vi "Install Dependencies.vi"(7 "Stored Install Data":path, 10 "Variant":variant) -> (0 "Error Out":errorcluster)   [LabVIEW 2020, in "LMH-Toolbox.lvlib" / "LMH-Installer Tools.lvlib"]
uses:
  LMH-Installer Tools.lvlib
  Private/Type Defs/Deps State.ctl
  <vilib>/Utility/file.llb/Read From Spreadsheet File (string).vi
  LMH-Toolbox.lvlib
panel:
  out "Tab Control":T1(tab)
  out "Package Name":string
  in  "Listbox":i32(listbox)
  in  "Info Cancel Button":bool
  in  "Info Next Button":bool
  out "Status":string
  out "Download Progress":u8(slide) scale=0.0..100.0
  in  "Multicolumn Listbox":i32(listbox)
  in  "Install Next":bool
  in  "Install Cancel":bool
  in  "Summary Finish":bool
  # "Testing Dependencies . . ."
  # "Select dependencies you want to install."
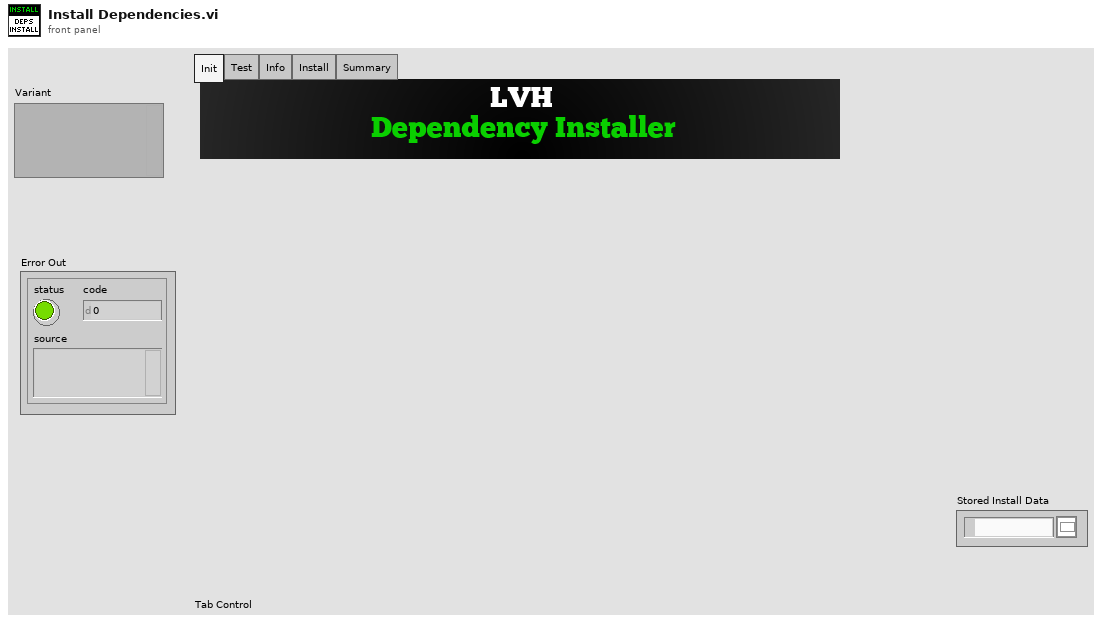
[diagram p1: front panel]
types:
  T1 = enum32{"Init", "Test", "Info", "Install", "Summary"}
  T2 = typedef "LMH-Toolbox.lvlib/LMH-Installer Tools.lvlib/Deps State.ctl" = enum16{"Init", "Test", "Info", "Install", "Summary"}
  T3 = typedef "LMH-Toolbox.lvlib/LMH-Installer Tools.lvlib/Dependency Config.ctl" = cluster{"Dependencies":T4[], "Files Installed":path[], "Dependency Config":path, "Installer Helper":path, "Dep Index":i32, "Download":T5}
  T4 = typedef "LMH-Toolbox.lvlib/LMH-Installer Tools.lvlib/Dependecy.ctl" = cluster{"Name":string, "Version":string, "Test VI Path":path, "Source URL":string, "Dep Met?":bool, "Install?":bool, "Installer Args":string}
  T5 = typedef "LMH-Toolbox.lvlib/LMH-Web.lvlib/Download Task.ctl" = cluster{"URL":string, "Local Path":path, "Download Worker":refnum<vi>, "Total Size (Bytes)":u64, "Prev Downloaded Size":u64, "Prev Download Time Stamp":timestamp}
  T6 = enum16{"Init", "Start DL", "Downloading", "DL Complete", "Done"}
  T7 = typedef "LVPoint32TypeDef.ctl" = cluster{"Horizontal":i32, "Vertical":i32}
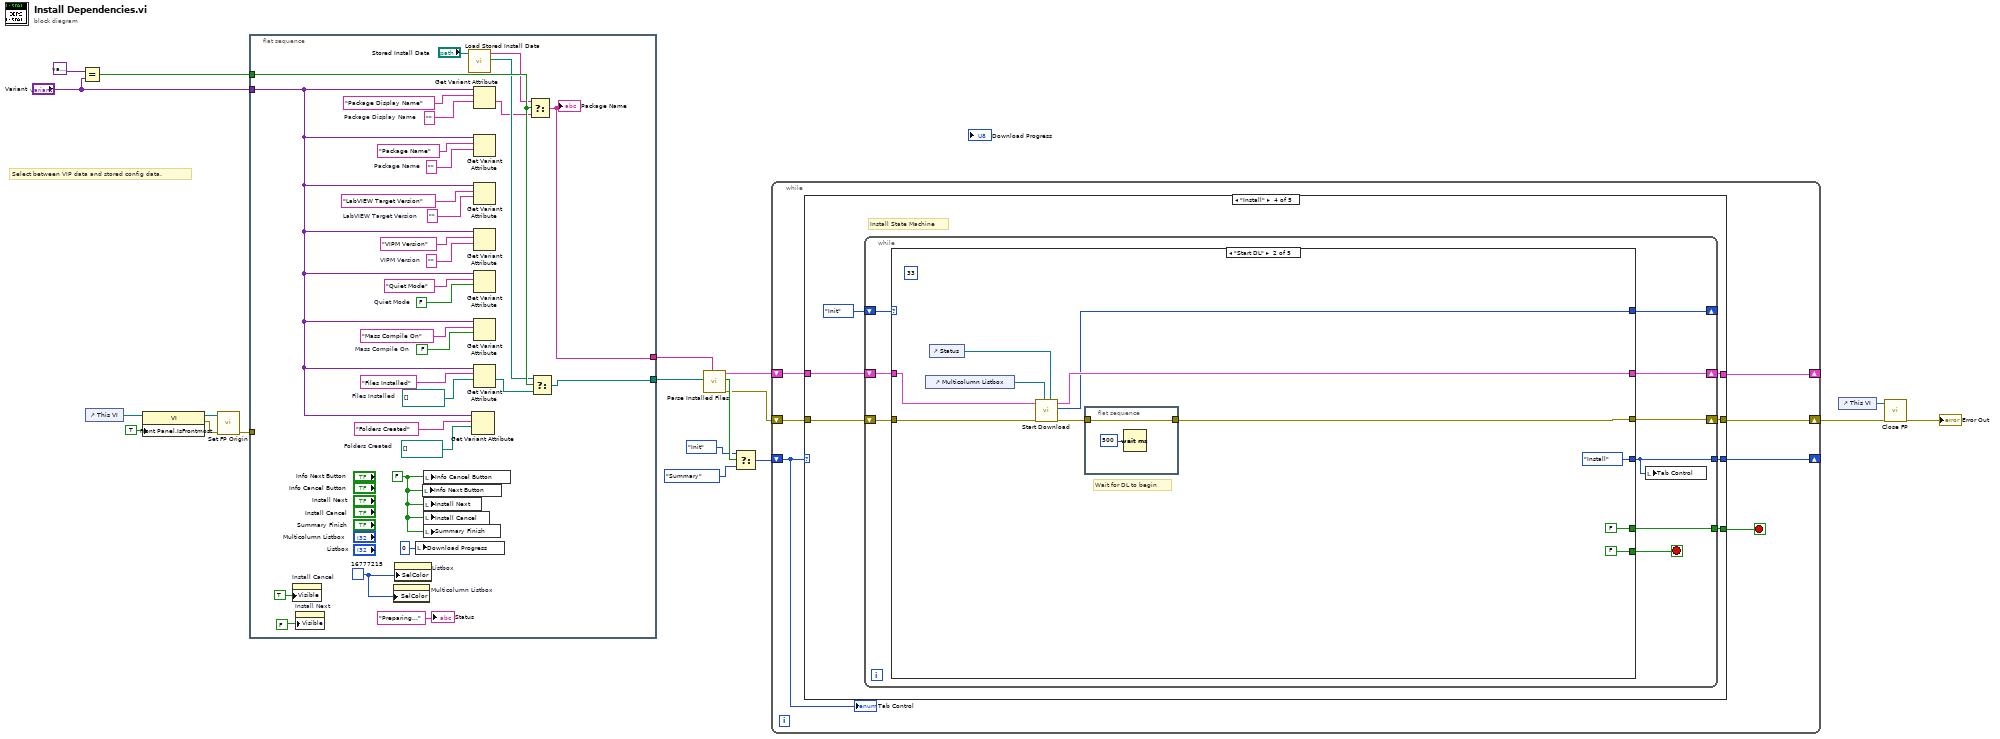
[diagram p0: block diagram]
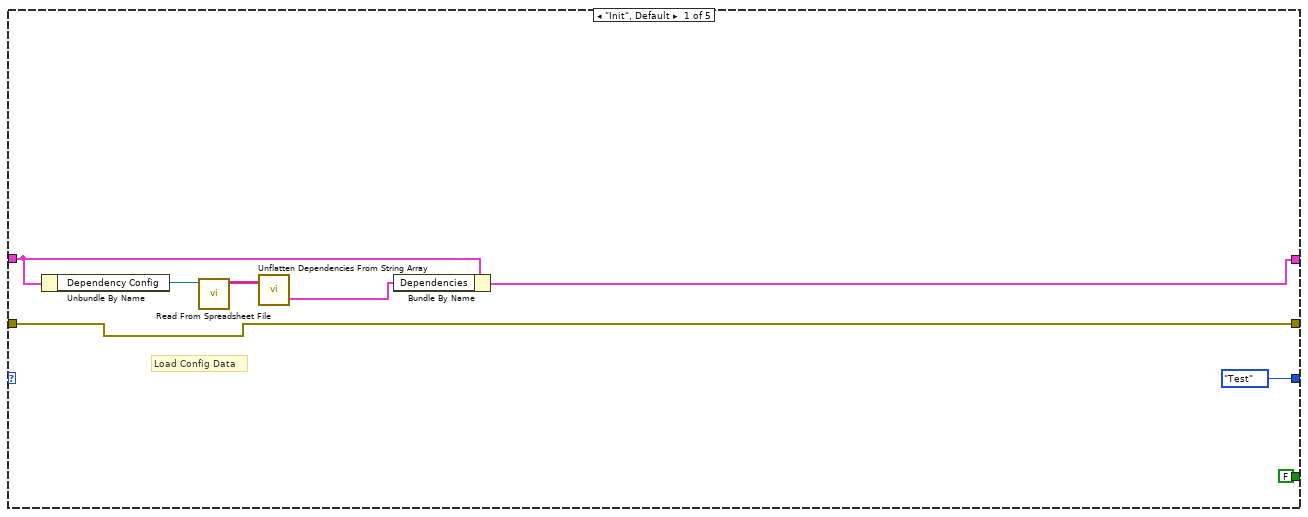
[diagram p2: hidden frame]
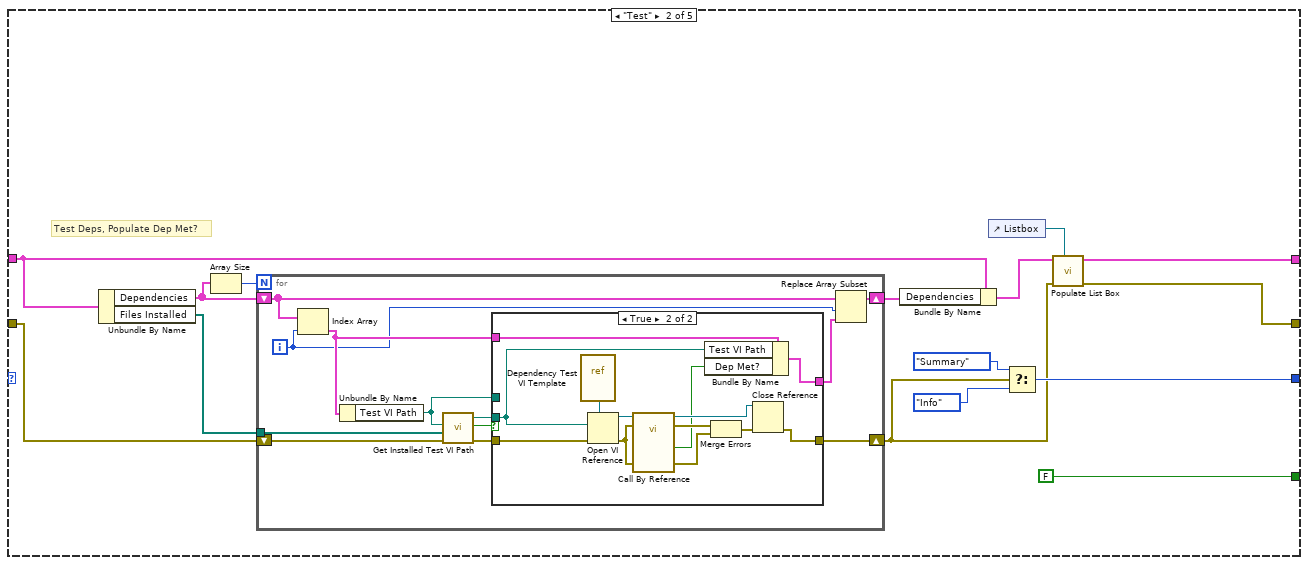
[diagram p3: hidden frame]
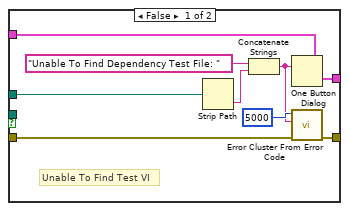
[diagram p4: hidden frame]
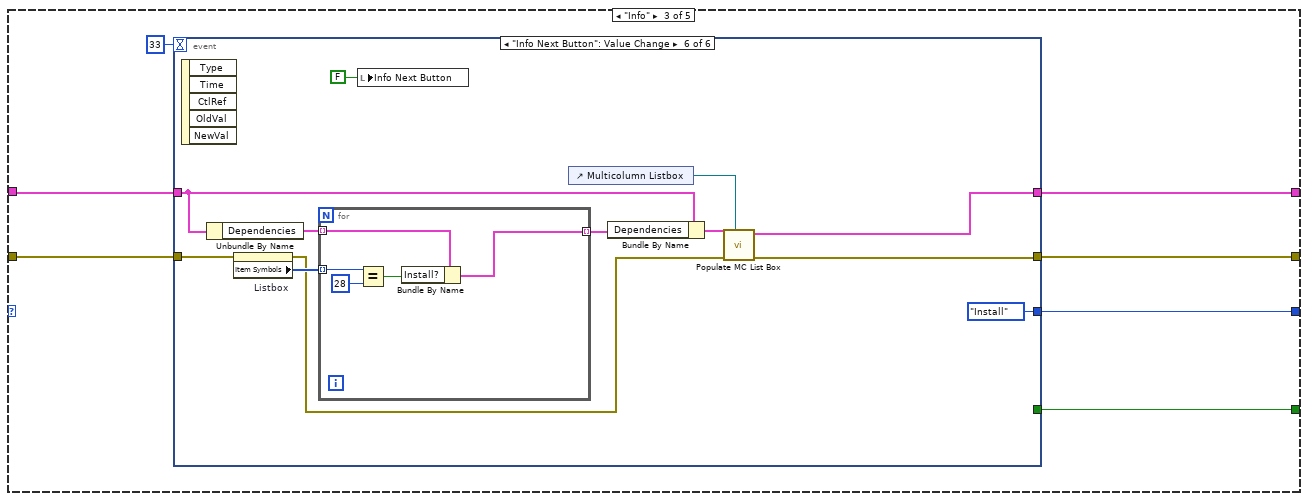
[diagram p5: hidden frame]
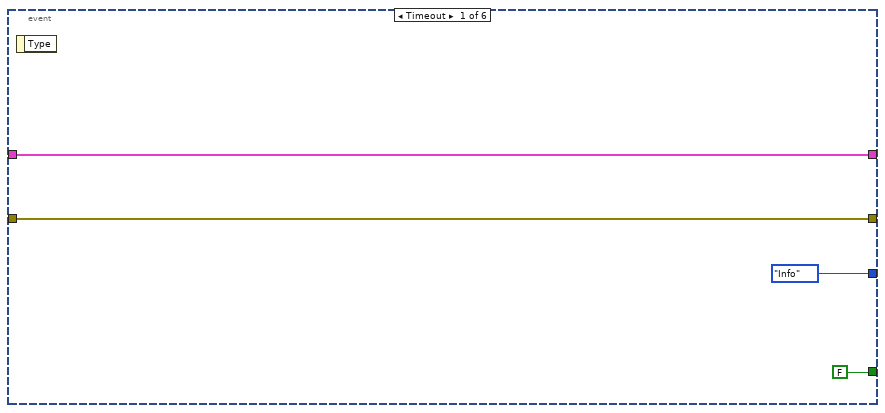
[diagram p6: hidden frame]
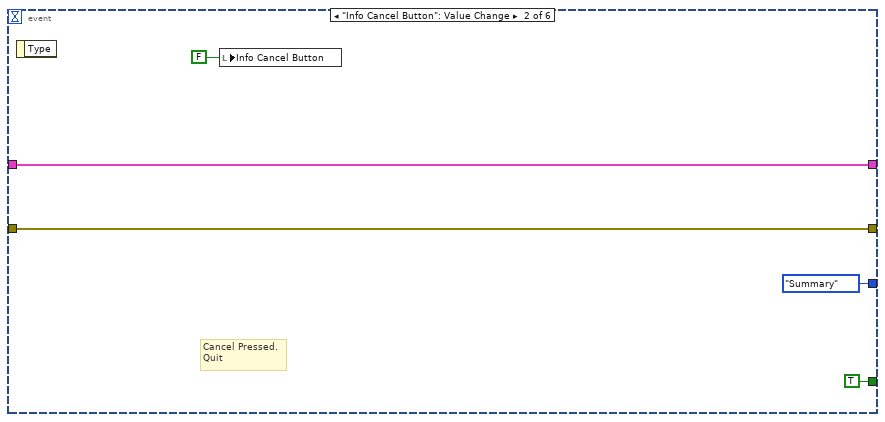
[diagram p7: hidden frame]
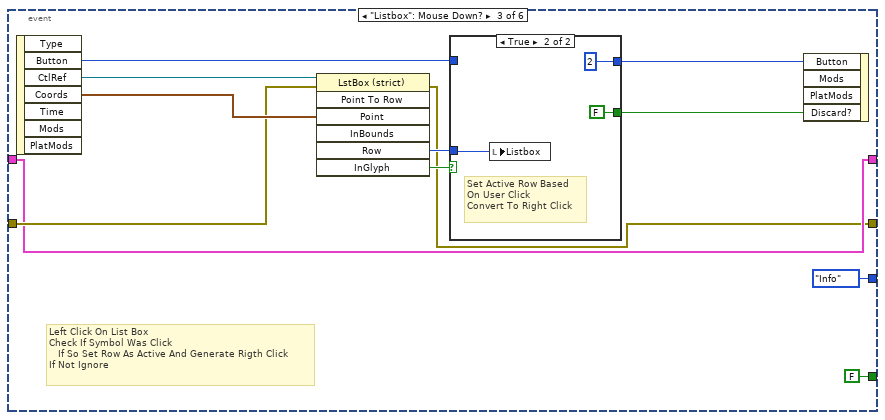
[diagram p8: hidden frame]
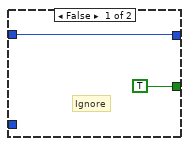
[diagram p9: hidden frame]
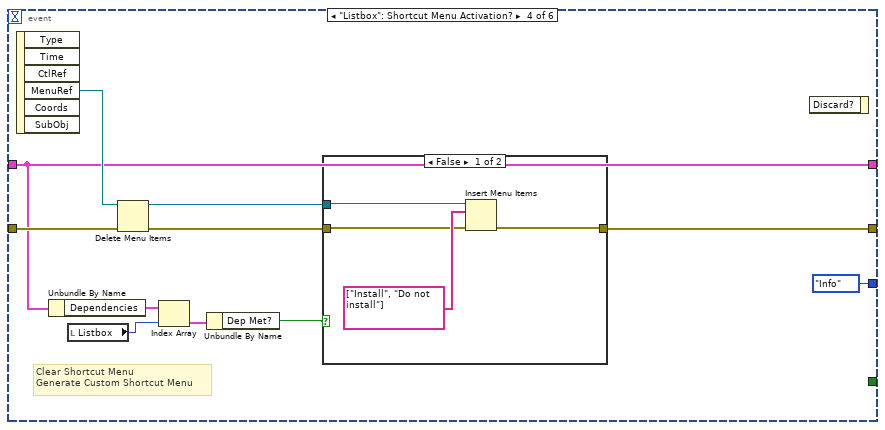
[diagram p10: hidden frame]
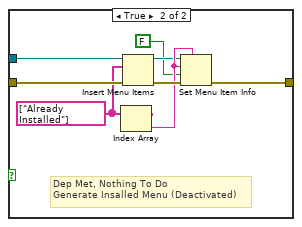
[diagram p11: hidden frame]
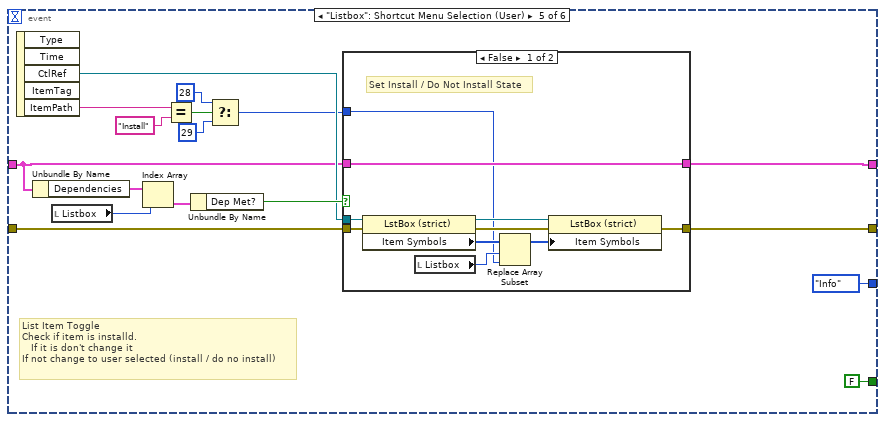
[diagram p12: hidden frame]
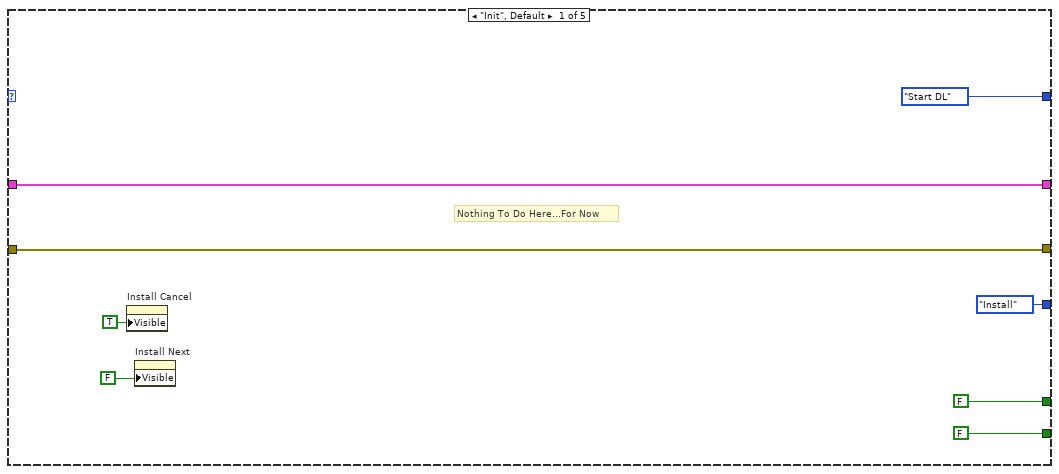
[diagram p14: hidden frame]
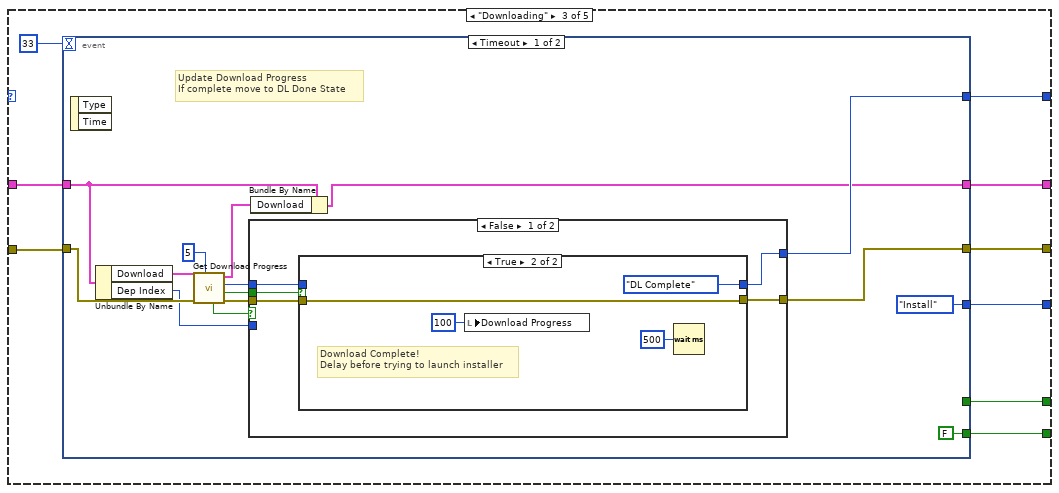
[diagram p15: hidden frame]
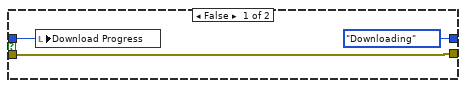
[diagram p16: hidden frame]
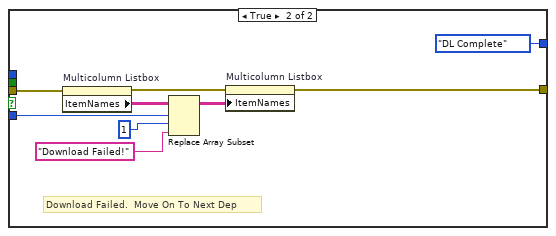
[diagram p17: hidden frame]
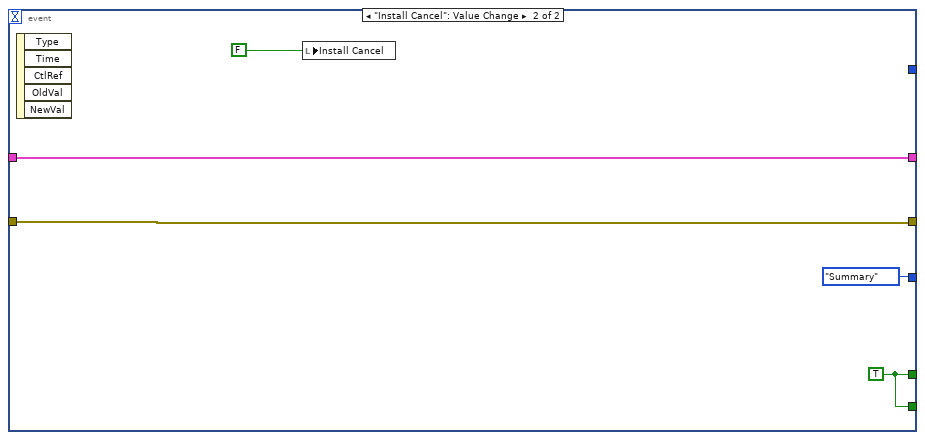
[diagram p18: hidden frame]
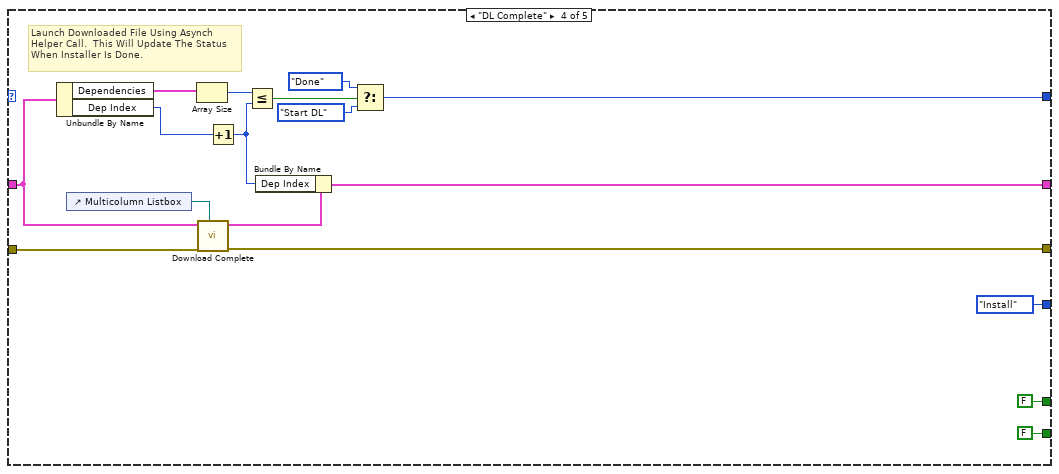
[diagram p19: hidden frame]
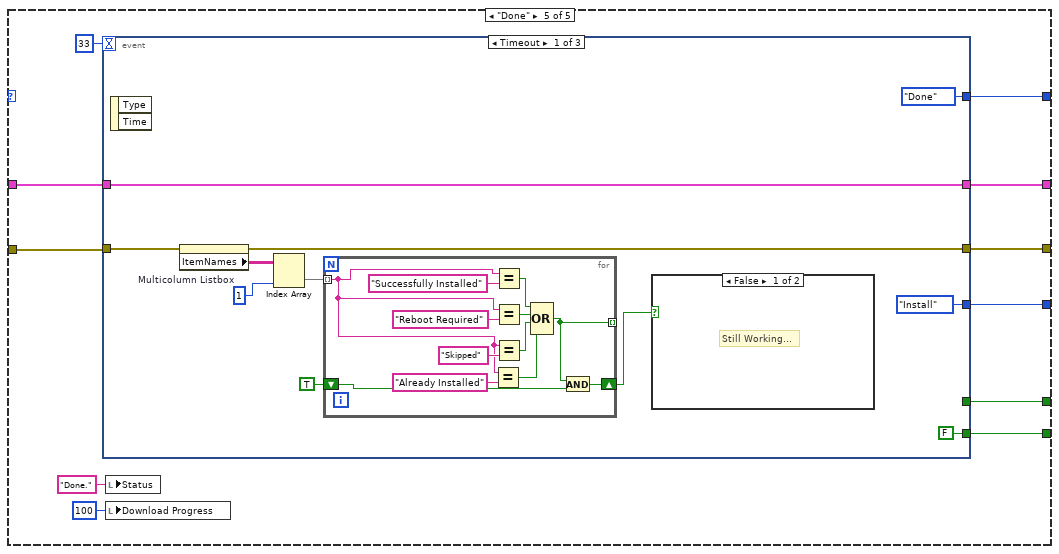
[diagram p20: hidden frame]
diagram:
  # "Select between VIP data and stored config data."
  n1 = Equal?(x=variant ("Variant"), y="Variant") -> (x = y?=w6:bool)
  n2 = control-ref of="This VI"() -> (w3:refnum<vi>)
  n3 = property class="VI"(reference=w3, "Front Panel.IsFrontmost"=TRUE ("Front Panel Window:Is Frontmost")) -> (reference out=w4:refnum<vi>, error out=w2:errorcluster)  [unwired: 1 in]
  n4 = call "Set FP Origin.vi"("Error In"=w2, "VI Ref"=w4) -> ("Error Out"=w14:errorcluster)  [unwired: 9 in]
  n5 = flat-sequence {
    tunnel: w14 -> [_]
    tunnel: "Variant" -> [w28]
    tunnel: [w24] -> w8
    tunnel: w6 -> [w27]
    tunnel: [w25] -> w5
    frame #0 {
      w34 = u32 16777215
      w32 = FALSE ("Cancel Button")
      w35 = path[] []  # Folders Created
      w36 = path[] []  # Files Installed
      w39 = FALSE  # Mass Compile On
      w40 = ""  # Package Display Name
      w41 = FALSE  # Quiet Mode
      w44 = ""  # VIPM Version
      w46 = ""  # LabVIEW Target Version
      w48 = ""  # Package Name
      n6 = property on="Install Cancel" class="Bool (strict)"("Visible"=TRUE) -> ()  [unwired: 2 in, 2 out]
      n7 = property on="Install Next" class="Bool (strict)"("Visible"=FALSE) -> ()  [unwired: 2 in, 2 out]
      n8 = property on="Multicolumn Listbox" class="MCListbox (strict)"("SelColor"=w34) -> ()  [unwired: 2 in, 2 out]
      n9 = property on="Listbox" class="LstBox (strict)"("SelColor"=w34) -> ()  [unwired: 2 in, 2 out]
      n10 = local write "Download Progress"(u8 0 ("Download Progress")) -> ()
      n11 = local write "Info Next Button"(w32) -> ()
      n12 = local write "Info Cancel Button"(w32) -> ()
      n13 = local write "Install Next"(w32) -> ()
      n14 = local write "Install Cancel"(w32) -> ()
      n15 = local write "Summary Finish"(w32) -> ()
      n16 = call "Load Stored Install Data.vi"("Stored Install Data"="Stored Install Data") -> ("Installed Files"=w23:path[], "Package Display Name"=w21:string)  [unwired: 9 in]
      n17 = Get Variant Attribute(Variant=w28, name="Folders Created", default value (empty Variant)=w35) -> ()  [unwired: 1 in, 4 out]
      n18 = Get Variant Attribute(Variant=w28, name="Package Display Name", default value (empty Variant)=w40) -> (value=w20:string)  [unwired: 1 in, 3 out]
      n19 = Get Variant Attribute(Variant=w28, name="Package Name", default value (empty Variant)=w48) -> ()  [unwired: 1 in, 4 out]
      n20 = Get Variant Attribute(Variant=w28, name="LabVIEW Target Version", default value (empty Variant)=w46) -> ()  [unwired: 1 in, 4 out]
      n21 = Get Variant Attribute(Variant=w28, name="VIPM Version", default value (empty Variant)=w44) -> ()  [unwired: 1 in, 4 out]
      n22 = Get Variant Attribute(Variant=w28, name="Quiet Mode", default value (empty Variant)=w41) -> ()  [unwired: 1 in, 4 out]
      n23 = Get Variant Attribute(Variant=w28, name="Mass Compile On", default value (empty Variant)=w39) -> ()  [unwired: 1 in, 4 out]
      n24 = Get Variant Attribute(Variant=w28, name="Files Installed", default value (empty Variant)=w36) -> (value=w22:path[])  [unwired: 1 in, 3 out]
      n25 = Select(t=w21, s=w27, f=w20) -> (s? t:f=w24:string)
      "Package Name" <- w24
      n26 = Select(t=w23, s=w27, f=w22) -> (s? t:f=w25:path[])
      "Status" <- "Preparing..." ("Status")
    }
  }
  n27 = call "Parse Installed Files.vi"("Package Name"=w8, "Files Installed"=w5) -> ("Error Out"=w13:errorcluster, "Config Found?"=w19:bool, "Dependecy Config out"=w15:T3)  [unwired: 7 in]
  n28 = Select(t=Deps_State."Init" ("Deps State"), s=w19, f=Deps_State."Summary" ("Deps State")) -> (s? t:f=w16:T2)
  n29 = while {
    shift-right: [w53] -> _
    shift-left: w16 -> [w51]
    shift-right: [w57] -> _
    shift-left: w15 -> [w56]
    shift-right: [w54] -> w11
    shift-left: w13 -> [w55]
    stop <- w52 stop-if-true
    n30 = case shown="\"Install\"" w51 {
      tunnel: [w64 w69 w115 w219 w371] -> w57
      tunnel: w56 -> [w63 w76 w120 w222 w370]
      tunnel: w55 -> [w61 w79 w118 w221 w373]
      tunnel: [w61 w66 w119 w220 w372] -> w54
      tunnel: [Deps_State."Test" ("Deps State") w72 w117 w216 Deps_State."Summary" ("Deps State")] -> w53
      tunnel: [FALSE FALSE w116 w217 w374] -> w52
      frame "Init", Default {
        # "Load Config Data"
        n31 = Unbundle By Name(w63) -> ("Dependency Config"=w62:path)
        n32 = call-poly <vilib>:"Read From Spreadsheet File.vi"("file path (dialog if empty)"=w62) -> ("all rows"=w65:string[][])  [unwired: 6 in, 4 out]
        n33 = call "Unflatten Dependencies From String Array.vi"("Flattened Dependencies"=w65) -> ("Deps"=w58:T4[])  [unwired: 1 in, 1 out]
        n34 = Bundle By Name(cluster=w63, "Dependencies"=w58) -> (w64:T3)
      }
      frame "Test" {
        # "Test Deps, Populate Dep Met?"
        n35 = Unbundle By Name(w76) -> ("Dependencies"=w77:T4[], "Files Installed"=w80:path[])
        n36 = Array Size(array=w77) -> (size(s)=w78:i32)
        n37 = for {
          N: w78 -> [_]
          tunnel: w80 -> [w92]
          shift-right: [w83] -> w68
          shift-left: w79 -> [w91]
          shift-right: [w86] -> w75
          shift-left: w77 -> [w85]
          i -> [w82]
          n38 = Index Array(array=w85, index=w82) -> (element=w87:T4)
          n39 = Unbundle By Name(w87) -> ("Test VI Path"=w81:path)
          n40 = call "Get Installed Test VI Path.vi"("Error In"=w91, "Files Installed"=w92, "Test VI Path"=w81) -> ("Error Out"=w90:errorcluster, "Found?"=w88:bool, "Installed Test VI Path"=w89:path)  [unwired: 6 in]
          n41 = case shown="True" w88 {
            tunnel: w90 -> [w98 w113]
            tunnel: w89 -> [_ w101]
            tunnel: [w100 w104] -> w84
            tunnel: w87 -> [w100 w103]
            tunnel: [w97 w102] -> w83
            tunnel: w81 -> [w93 _]
            frame False {
              # "Unable To Find Test VI"
              n42 = Strip Path(path=w93) -> (name=w95:string)  [unwired: 1 out]
              n43 = Concatenate Strings("Unable To Find Dependency Test File: " ("message"), w95) -> (w94:string)
              n44 = One Button Dialog(message=w94) -> ()  [unwired: 1 in, 1 out]
              n45 = call <vilib>:"Error Cluster From Error Code.vi"("error in (no error)"=w98, "error message (\"\")"=w94, "error code (0)"=5000) -> ("error out"=w97:errorcluster)  [unwired: 6 in]
            }
            frame True {
              n46 = vi-ref "Dependency Test VI Template.vi"() -> (w111:refnum<vi>)
              n47 = Open VI Reference(type specifier VI Refnum (for type only)=w111, vi path=w101, error in (no error)=w113) -> (vi reference=w112:refnum<vi>, error out=w110:errorcluster)  [unwired: 3 in]
              n48 = call-by-ref "?"(reference=w112, error in=w110, "Error In"=w110) -> (reference out=w106:refnum<vi>, error out=w109:errorcluster, "Error Out"=w108:errorcluster, "Pass?"=w105:bool)  [unwired: 9 in]
              n49 = Bundle By Name(cluster=w103, "Test VI Path"=w101, "Dep Met?"=w105) -> (w104:T4)
              n50 = Merge Errors(w109, w108) -> (w107:errorcluster)
              n51 = Close Reference(reference=w106, error in (no error)=w107) -> (error out=w102:errorcluster)
            }
          }
          n52 = Replace Array Subset(array=w85, new element=w84, index=w82) -> (w86:T4[])
        }
        n53 = Bundle By Name(cluster=w76, "Dependencies"=w75) -> (w70:T3)
        n54 = control-ref of="Listbox"() -> (w67:refnum<vi>)
        n55 = Select(t=Deps_State."Summary" ("Deps State"), s=w68, f=Deps_State."Info" ("Deps State")) -> (s? t:f=w72:T2)
        n56 = call "Populate List Box.vi"("Listbox Ref"=w67, "Error In"=w68, "Dependecy Config"=w70) -> ("Error Out"=w66:errorcluster, "Dependecy Config"=w69:T3)  [unwired: 7 in]
      }
      frame "Info" {
        n57 = event shown="[5] \"Info Next Button\": Value Change" {
          selector: _ -> [_ _ _ _ _ _]
          dyn-events: _ -> [_ _ _ _ _ _]
          timeout: 33 -> [_ _ _ _ _ _]
          tunnel: w120 -> [w121 w125 w133 w149 w171 w203]
          tunnel: [w122 w126 w131 w148 w173 w199] -> w119
          tunnel: w118 -> [w122 w126 w139 w157 w178 w204]
          tunnel: [Deps_State."Info" ("Deps State") Deps_State."Summary" ("Deps State") Deps_State."Info" ("Deps State") Deps_State."Info" ("Deps State") Deps_State."Info" ("Deps State") Deps_State."Install" ("Deps State")] -> w117
          tunnel: [FALSE TRUE FALSE _ FALSE _] -> w116
          tunnel: [w121 w125 w133 w149 w172 w208] -> w115
          event Timeout {
            n58 = event-data() -> ()  [unwired: 1 in, 1 out]
          }
          event "Info Cancel Button": Value Change {
            # "Cancel Pressed.\nQuit"
            n59 = event-data() -> ()  [unwired: 1 in, 1 out]
            n60 = local write "Info Cancel Button"(FALSE ("Cancel Button")) -> ()
          }
          event "Listbox": Mouse Down? {
            # "Left Click On List Box\nCheck If Symbol Was Click\n   If So Set Row As Active And Generate Rigth Click\nIf Not Ignore"
            n61 = event-data() -> ("Button"=w134:u16, "CtlRef"=w141:refnum<vi>, "Coords"=w140:T7)  [unwired: 1 in, 4 out]
            n62 = invoke class="LstBox (strict)" method="Point To Row"(reference=w141, error in=w139, "Point"=w140) -> (error out=w131:errorcluster, "Row"=w136:i32, "InGlyph"=w138:bool)  [unwired: 4 in, 4 out]
            n63 = case shown="True" w138 {
              tunnel: w136 -> [_ w145]
              tunnel: [w143 u16 2 ("Button")] -> w135
              tunnel: w134 -> [w143 _]
              tunnel: [TRUE FALSE] -> w130
              frame False {
                # "Ignore"
              }
              frame True {
                # "Set Active Row Based \nOn User Click\nConvert To Right Click"
                n64 = local write "Listbox"(w145) -> ()
              }
            }
            n65 = event-data("Button"=w135, "Discard?"=w130) -> ()  [unwired: 3 in, 1 out]
          }
          event "Listbox": Shortcut Menu Activation? {
            # "Clear Shortcut Menu\nGenerate Custom Shortcut Menu"
            n66 = event-data() -> ("MenuRef"=w156:refnum<k9>)  [unwired: 1 in, 5 out]
            n67 = Unbundle By Name(w149) -> ("Dependencies"=w152:T4[])
            n68 = local read "Listbox"() -> (w151:i32)
            n69 = Delete Menu Items(6:w157, 9:w156) -> (0:w154:errorcluster, 3:w153:refnum<k9>)  [unwired: 2 in]
            n70 = Index Array(array=w152, index=w151) -> (element=w150:T4)
            n71 = Unbundle By Name(w150) -> ("Dep Met?"=w147:bool)
            n72 = case shown="False" w147 {
              tunnel: w154 -> [w160 w169]
              tunnel: w153 -> [w159 w168]
              tunnel: [w158 w166] -> w148
              frame False {
                n73 = Insert Menu Items(6:w160, 8:string[] ["Install", "Do not install"], 9:w159) -> (0:w158:errorcluster)  [unwired: 3 in, 2 out]
              }
              frame True {
                w165 = string[] ["Already Installed"] ("item names")
                # "Dep Met, Nothing To Do\nGenerate Insalled Menu (Deactivated)"
                n74 = Index Array(array=w165) -> (element=w164:string)  [unwired: 1 in]
                n75 = Insert Menu Items(6:w169, 8:w165, 9:w168) -> (0:w167:errorcluster, 3:w163:refnum<k9>)  [unwired: 3 in, 1 out]
                n76 = Set Menu Item Info(7:w164, 8:w167, 9:FALSE ("enabled"), 10:w164, 11:w163) -> (0:w166:errorcluster)  [unwired: 2 in, 1 out]
              }
            }
            n77 = event-data() -> ()  [unwired: 2 in, 1 out]
          }
          event "Listbox": Shortcut Menu Selection (User) {
            # "List Item Toggle\nCheck if item is installd.\n   If it is don't change it\nIf not change to user selected (install / do no install)"
            n78 = event-data() -> ("CtlRef"=w179:refnum<vi>, "ItemPath"=w185:string)  [unwired: 1 in, 3 out]
            n79 = Unbundle By Name(w171) -> ("Dependencies"=w183:T4[])
            n80 = local read "Listbox"() -> (w182:i32)
            n81 = Index Array(array=w183, index=w182) -> (element=w181:T4)
            n82 = Equal?(x=w185, y="Install") -> (x = y?=w177:bool)
            n83 = Unbundle By Name(w181) -> ("Dep Met?"=w180:bool)
            n84 = Select(t=28, s=w177, f=29 ("t")) -> (s? t:f=w174:i32)
            n85 = case shown="False" w180 {
              tunnel: w179 -> [w196 _]
              tunnel: w178 -> [w195 w198]
              tunnel: w174 -> [w187 _]
              tunnel: [w190 w198] -> w173
              tunnel: [w189 w197] -> w172
              tunnel: w171 -> [w189 w197]
              frame False {
                # "Set Install / Do Not Install State"
                n86 = property class="LstBox (strict)"(reference=w196, error in=w195) -> (reference out=w194:refnum<vi>, error out=w193:errorcluster, "Item Symbols"=w192:i32[])
                n87 = local read "Listbox"() -> (w188:i32)
                n88 = Replace Array Subset(array=w192, new element=w187, index=w188) -> (w191:i32[])
                n89 = property class="LstBox (strict)"(reference=w194, error in=w193, "Item Symbols"=w191) -> (error out=w190:errorcluster)  [unwired: 1 out]
              }
              frame True {
                # "Dependency is installd.   Leave it alone."
              }
            }
          }
          event "Info Next Button": Value Change {
            n90 = event-data() -> ()  [unwired: 1 in, 5 out]
            n91 = Unbundle By Name(w203) -> ("Dependencies"=w206:T4[])
            n92 = property on="Listbox" class="LstBox (strict)"(error in=w204) -> (error out=w200:errorcluster, "Item Symbols"=w205:i32[])  [unwired: 1 in, 1 out]
            n93 = for {
              tunnel: w206 -> [w212] mode=indexing
              tunnel: w205 -> [w214] mode=indexing
              tunnel: [w211] -> w202 mode=indexing
              n94 = Equal?(x=w214, y=28) -> (x = y?=w213:bool)
              n95 = Bundle By Name(cluster=w212, "Install?"=w213) -> (w211:T4)
            }
            n96 = local write "Info Next Button"(FALSE ("Next Button")) -> ()
            n97 = control-ref of="Multicolumn Listbox"() -> (w207:refnum<vi>)
            n98 = Bundle By Name(cluster=w203, "Dependencies"=w202) -> (w201:T3)
            n99 = call "Populate MC List Box.vi"("Listbox Ref"=w207, "Error In"=w200, "Dependecy Config"=w201) -> ("Error Out"=w199:errorcluster, "Dependecy Config"=w208:T3)  [unwired: 7 in]
          }
        }
      }
      frame "Install" {
        # "Install State Machine"
        n100 = while {
          shift-right: [w224] -> _
          shift-left: T6."Init" ("Install State") -> [w226]
          tunnel: [w225] -> w217
          tunnel: [w223] -> w216
          shift-right: [w228] -> w219
          shift-left: w222 -> [w231]
          shift-right: [w229] -> w220
          shift-left: w221 -> [w230]
          stop <- w227 stop-if-true
          n101 = case shown="\"Start DL\"" w226 {
            tunnel: w231 -> [w236 w245 w261 w310 w330]
            tunnel: w230 -> [w237 w250 w260 w316 w323]
            tunnel: [w237 w241 w259 w317 w329] -> w229
            tunnel: [w236 w244 w258 w306 w328] -> w228
            tunnel: [FALSE FALSE w256 FALSE w326] -> w227
            tunnel: [FALSE FALSE w255 FALSE w325] -> w225
            tunnel: [Deps_State."Install" ("Deps State") Deps_State."Install" ("Deps State") w254 Deps_State."Install" ("Deps State") w324] -> w223
            tunnel: [T6."Start DL" ("Install State") w243 w253 w305 w320] -> w224
            frame "Init", Default {
              # "Nothing To Do Here...For Now"
              n102 = property on="Install Cancel" class="Bool (strict)"("Visible"=TRUE) -> ()  [unwired: 2 in, 2 out]
              n103 = property on="Install Next" class="Bool (strict)"("Visible"=FALSE) -> ()  [unwired: 2 in, 2 out]
            }
            frame "Start DL" {
              (unwired) 33
              # "Wait for DL to begin"
              n104 = control-ref of="Multicolumn Listbox"() -> (w246:refnum<vi>)
              n105 = control-ref of="Status"() -> (w247:refnum<vi>)
              n106 = call "Start Download.vi"("Overall Status"=w247, "Itemized Status"=w246, "Error In"=w250, "Dependecy Config"=w245) -> ("Error Out"=w240:errorcluster, "Install State"=w243:T6, "Dependecy Config"=w244:T3)  [unwired: 5 in]
              n107 = flat-sequence {
                tunnel: [w251] -> w241
                tunnel: w240 -> [w251]
                frame #0 {
                  n108 = Wait (ms)(milliseconds to wait=u32 500) -> ()  [unwired: 1 out]
                }
              }
            }
            frame "Downloading" {
              n109 = event shown="[0] Timeout" {
                selector: _ -> [_ _]
                dyn-events: _ -> [_ _]
                timeout: 33 -> [_ _]
                tunnel: w261 -> [w265 w299]
                tunnel: [w271 w298] -> w259
                tunnel: w260 -> [w275 w298]
                tunnel: [FALSE w301] -> w256
                tunnel: [w264 w299] -> w258
                tunnel: [_ w301] -> w255
                tunnel: [Deps_State."Install" ("Deps State") Deps_State."Summary" ("Deps State")] -> w254
                tunnel: [w269 _] -> w253
                event Timeout {
                  # "Update Download Progress\nIf complete move to DL Done State"
                  n110 = event-data() -> ()  [unwired: 1 in, 2 out]
                  n111 = Unbundle By Name(w265) -> ("Download"=w267:T5, "Dep Index"=w263:i32)
                  n112 = call "Get Download Progress.vi"("Download Timeout (S)"=u32 5, "Error In"=w275, "Download"=w267) -> ("Error Out"=w272:errorcluster, "Complete?"=w270:bool, "Percent Complete"=w268:i32, "Download"=w266:T5, "Timeout?"=w273:bool)  [unwired: 4 in]
                  n113 = case shown="False" w273 {
                    tunnel: w272 -> [w279 w297]
                    tunnel: [w278 w292] -> w271
                    tunnel: w270 -> [w281 _]
                    tunnel: [w280 T6."DL Complete" ("Install State")] -> w269
                    tunnel: w268 -> [w277 _]
                    tunnel: w263 -> [_ w289]
                    frame False {
                      n114 = case shown="True" w281 {
                        tunnel: [T6."Downloading" ("Install State") T6."DL Complete" ("Install State")] -> w280
                        tunnel: w279 -> [w283 w286]
                        tunnel: [w283 w286] -> w278
                        tunnel: w277 -> [w284 _]
                        frame False {
                          n115 = local write "Download Progress"(w284) -> ()
                        }
                        frame True {
                          # "Download Complete!\nDelay before trying to launch installer"
                          n116 = local write "Download Progress"(u8 100 ("Download Progress")) -> ()
                          n117 = Wait (ms)(milliseconds to wait=u32 500) -> ()  [unwired: 1 out]
                        }
                      }
                    }
                    frame True {
                      # "Download Failed.  Move On To Next Dep"
                      n118 = property on="Multicolumn Listbox" class="MCListbox (strict)"(error in=w297) -> (error out=w294:errorcluster, "ItemNames"=w296:string[][])  [unwired: 1 in, 1 out]
                      n119 = Replace Array Subset(array=w296, new element="Download Failed!" ("new element/subarray"), index (row)=w289, index (col)=1 ("disabled index (col)")) -> (w293:string[][])
                      n120 = property on="Multicolumn Listbox" class="MCListbox (strict)"(error in=w294, "ItemNames"=w293) -> (error out=w292:errorcluster)  [unwired: 1 in, 1 out]
                    }
                  }
                  n121 = Bundle By Name(cluster=w265, "Download"=w266) -> (w264:T3)
                }
                event "Install Cancel": Value Change {
                  w301 = TRUE
                  n122 = event-data() -> ()  [unwired: 1 in, 5 out]
                  n123 = local write "Install Cancel"(FALSE ("Cancel Button")) -> ()
                }
              }
            }
            frame "DL Complete" {
              # "Launch Downloaded File Using Asynch\nHelper Call.  This Will Update The Status\nWhen Installer Is Done."
              n124 = Unbundle By Name(w310) -> ("Dependencies"=w309:T4[], "Dep Index"=w308:i32)
              n125 = control-ref of="Multicolumn Listbox"() -> (w315:refnum<vi>)
              n126 = Array Size(array=w309) -> (size(s)=w311:i32)
              n127 = call "Download Complete.vi"("MulticolumnListbox in"=w315, "Error In"=w316, "Dependency Config"=w310) -> ("Error Out"=w317:errorcluster, "Dependency Config"=w307:T3)  [unwired: 7 in]
              n128 = Increment(x=w308) -> (x+1=w304:i32)
              n129 = Less Or Equal?(x=w311, y=w304) -> (x <= y?=w314:bool)
              n130 = Bundle By Name(cluster=w307, "Dep Index"=w304) -> (w306:T3)
              n131 = Select(t=T6."Done" ("Install State"), s=w314, f=T6."Start DL" ("Install State")) -> (s? t:f=w305:T6)
            }
            frame "Done" {
              n132 = event shown="[0] Timeout" {
                selector: _ -> [_ _ _]
                dyn-events: _ -> [_ _ _]
                timeout: 33 -> [_ _ _]
                tunnel: w330 -> [w337 w359 w366]
                tunnel: [w336 w361 w367] -> w329
                tunnel: w323 -> [w338 w361 w367]
                tunnel: [FALSE TRUE w365] -> w326
                tunnel: [w337 w359 w366] -> w328
                tunnel: [_ TRUE w365] -> w325
                tunnel: [Deps_State."Install" ("Deps State") Deps_State."Summary" ("Deps State") Deps_State."Summary" ("Deps State")] -> w324
                tunnel: [T6."Done" ("Install State") T6."Done" ("Install State") T6."Done" ("Install State")] -> w320
                event Timeout {
                  n133 = event-data() -> ()  [unwired: 1 in, 2 out]
                  n134 = property on="Multicolumn Listbox" class="MCListbox (strict)"(error in=w338) -> (error out=w336:errorcluster, "ItemNames"=w335:string[][])  [unwired: 1 in, 1 out]
                  n135 = Index Array(array=w335, index (col)=1 ("index (row)")) -> (element=w334:string[])  [unwired: 1 in]
                  n136 = for {
                    tunnel: w334 -> [w343] mode=indexing
                    tunnel: [w349] -> _ mode=indexing
                    shift-right: [w348] -> w332
                    shift-left: TRUE -> [w347]
                    n137 = Equal?(x=w343, y="Already Installed") -> (x = y?=w342:bool)
                    n138 = Equal?(x=w343, y="Successfully Installed") -> (x = y?=w351:bool)
                    n139 = Equal?(x=w343, y="Reboot Required") -> (x = y?=w350:bool)
                    n140 = Equal?(x=w343, y="Skipped") -> (x = y?=w345:bool)
                    n141 = Compound Arithmetic op=OR(w351, w350, w345, w342) -> (w349:bool)
                    n142 = And(x=w349, y=w347) -> (x .and. y?=w348:bool)
                  }
                  n143 = case shown="False" w332 {
                    frame False {
                      # "Still Working..."
                    }
                    frame True {
                      # "Done"
                      n144 = property on="Install Cancel" class="Bool (strict)"("Visible"=FALSE) -> ()  [unwired: 2 in, 2 out]
                      n145 = property on="Install Next" class="Bool (strict)"("Visible"=TRUE) -> ()  [unwired: 2 in, 2 out]
                    }
                  }
                }
                event "Install Next": Value Change {
                  n146 = event-data() -> ()  [unwired: 1 in, 5 out]
                  n147 = local write "Install Next"(FALSE ("Next Button")) -> ()
                }
                event "Install Cancel": Value Change {
                  w365 = TRUE
                  n148 = event-data() -> ()  [unwired: 1 in, 5 out]
                  n149 = local write "Install Cancel"(FALSE ("Cancel Button")) -> ()
                }
              }
              n150 = local write "Status"("Done." ("Status")) -> ()
              n151 = local write "Download Progress"(u8 100 ("Download Progress")) -> ()
            }
          }
          n152 = local write "Tab Control"(w223) -> ()
        }
      }
      frame "Summary" {
        n153 = event shown="[1] \"Summary Finish\": Value Change" {
          selector: _ -> [_ _]
          dyn-events: _ -> [_ _]
          timeout: 33 -> [_ _]
          tunnel: [FALSE TRUE] -> w374
          tunnel: w373 -> [w377 w380]
          tunnel: [w377 w380] -> w372
          tunnel: [w376 w379] -> w371
          tunnel: w370 -> [w376 w379]
          event Timeout {
            n154 = event-data() -> ()  [unwired: 1 in, 2 out]
          }
          event "Summary Finish": Value Change {
            n155 = event-data() -> ()  [unwired: 1 in, 5 out]
            n156 = local write "Summary Finish"(FALSE ("Cancel Button")) -> ()
          }
        }
      }
    }
    "Tab Control" <- w51
  }
  n157 = control-ref of="This VI"() -> (w12:refnum<vi>)
  n158 = call "Close FP.vi"("Error In"=w11, "VI Ref"=w12) -> ("Error Out"=→"Error Out":errorcluster)  [unwired: 9 in]
